vi "iWorx - Spirometer.vi"() -> ()   [LabVIEW 2012]
uses:
  <vilib>/DAQmx/read.llb/DAQmx Read (Analog 1D Wfm NChan 1Samp).vi
  <vilib>/DAQmx/create/channels.llb/DAQmx Create Channel (AI-Voltage-Basic).vi
  <vilib>/DAQmx/configure/timing.llb/DAQmx Timing (Sample Clock).vi
  <vilib>/DAQmx/miscellaneous.llb/DAQmx Fill In Error Info.vi
panel:
  in  "Reset Integral":bool=TRUE
  in  "Set Up":bool
  out "Offset":dbl
  out "Slope":dbl=26.4
  in  "Set SP2":bool
  in  "Set SP1":bool
  in  "Channel":u16(ring) items=["Channel 1", "Channel 2"]
  in  "Calibration Data":T1={"SP1 Voltage"=1.0, "SP2 Voltage"=0.0, "SP1 Pressure"=26.4, "SP2 Pressure"=0.0} {"SP2 Voltage" format="%#_g V"; "SP1 Voltage" format="%#_g V"}
  in  "Pause Button":bool
  in  "Snapshot":bool
  out "Processed Signal":dbl(knob) caption="Pressue (mm H2O)" scale=-200.0..200.0
  in  "stop":bool
  out "Waveform Chart":waveform(dbl)[](graph)
  in  "Clear Chart":bool
  in  "Open Log":bool
  in  "Autoscale Y":bool=TRUE
  out "Raw Signal":dbl(knob) scale=-10.0..10.0
  # "iWorx - Spirometer - Data Logger"
  # "Sensor Input"
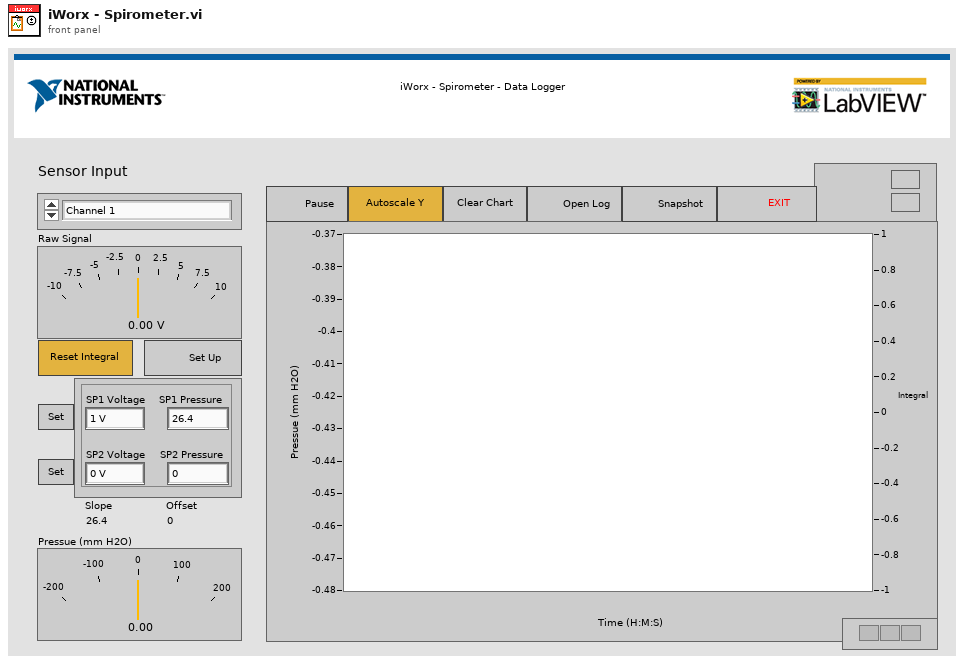
[diagram p1: front panel]
types:
  T1 = cluster{"SP1 Voltage":dbl, "SP2 Voltage":dbl, "SP1 Pressure":dbl, "SP2 Pressure":dbl}
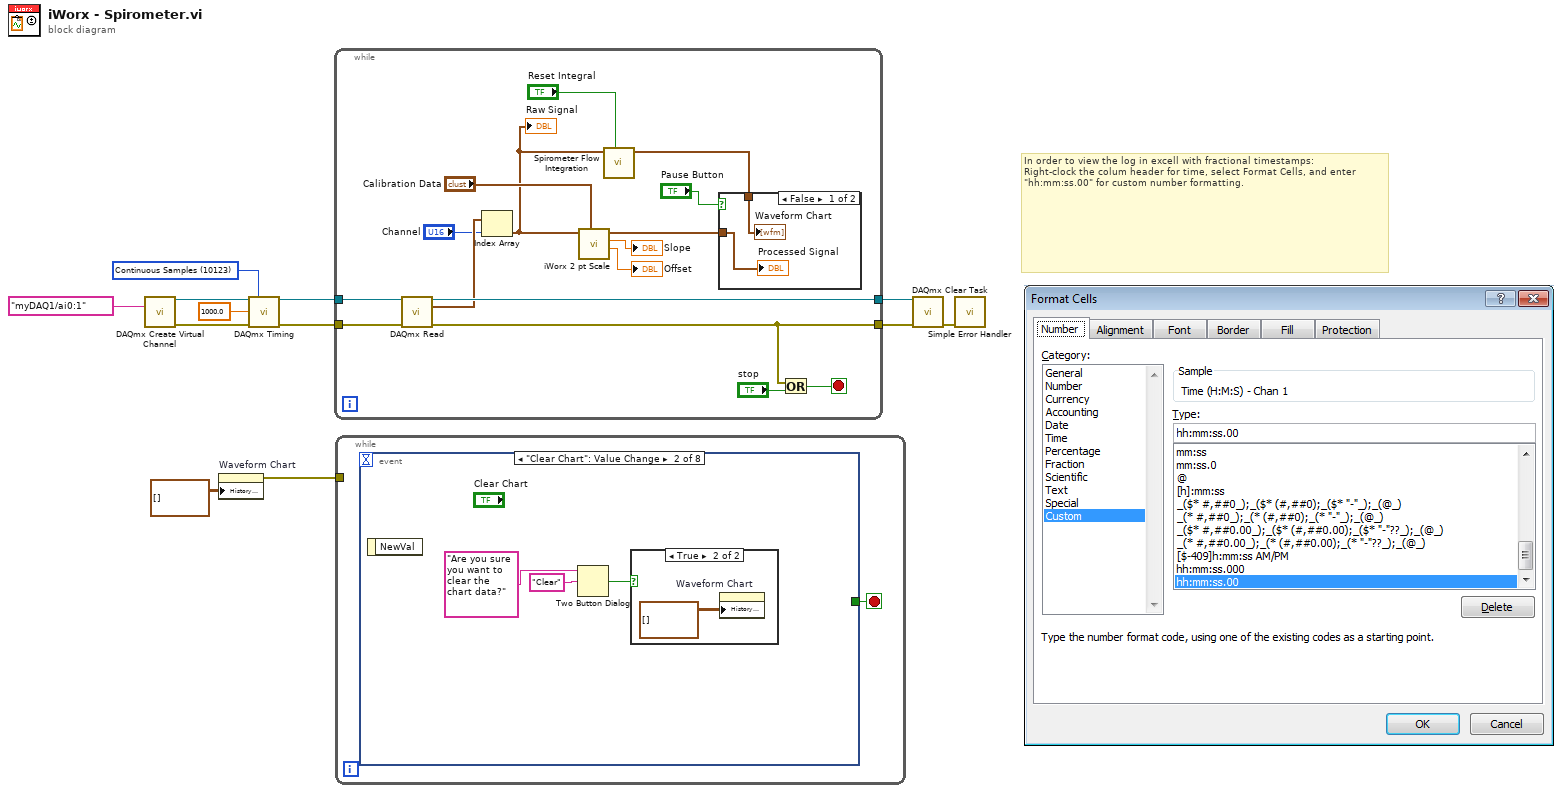
[diagram p0: block diagram]
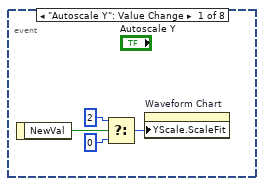
[diagram p2: hidden frame]
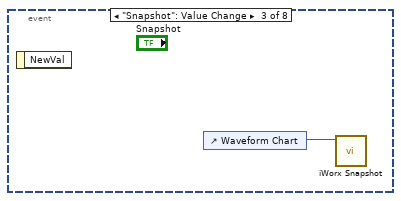
[diagram p4: hidden frame]
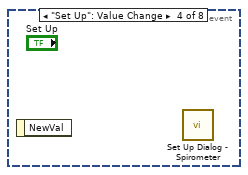
[diagram p5: hidden frame]
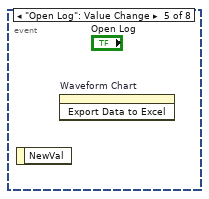
[diagram p6: hidden frame]
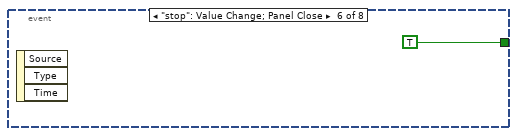
[diagram p7: hidden frame]
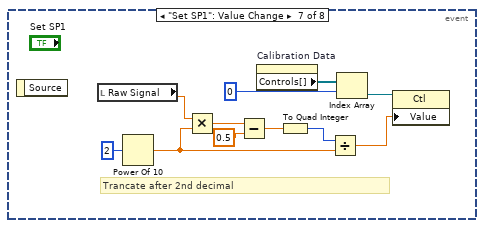
[diagram p8: hidden frame]
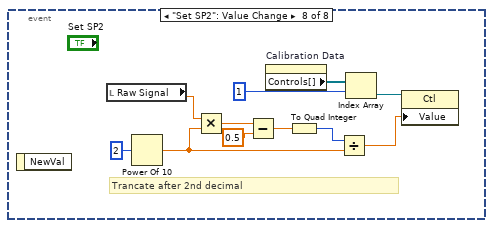
[diagram p9: hidden frame]
diagram:
  w2 = 10123 items=["Finite Samples"=10178, "Continuous Samples"=10123, "Hardware Timed Single Point"=12522] ("sample mode")
  # "In order to view the log in excell with fractional timestamps: \nRight-clock the colum header for time, select Format Cells, and enter \"hh:mm:ss.00\" for custom number formatting."
  n1 = call-poly <vilib>:"DAQmx Create Virtual Channel.vi"("physical channels"=tag "myDAQ1/ai0:1") -> ("task out"=w6:refnum<k21>, "error out"=w5:errorcluster)  [unwired: 13 in]
  n2 = property on="Waveform Chart" class="WFChart (strict)"("History Data"=waveform(dbl)[][] []) -> (error out=w9:errorcluster)  [unwired: 2 in, 1 out]
  n3 = call-poly <vilib>:"DAQmx Timing.vi"("task/channels in"=w6, "sample mode"=w2, "rate"=1000.0, "error in"=w5) -> ("task out"=w4:refnum<k21>, "error out"=w3:errorcluster)  [unwired: 10 in]
  n4 = while {
    tunnel: w4 -> [w27]
    tunnel: [w26] -> w12
    tunnel: w3 -> [w25]
    tunnel: [w23] -> w11
    stop <- w24 stop-if-true
    n5 = call-poly <vilib>:"DAQmx Read.vi"("task/channels in"=w27, "error in"=w25) -> ("task out"=w26:refnum<k21>, "data"=w21:waveform(dbl)[], "error out"=w23:errorcluster)  [unwired: 11 in]
    n6 = Index Array(array=w21, index="Channel") -> (element=w13:waveform(dbl))
    "Raw Signal" <- w13
    n7 = call "iWorx 2 pt Scale.vi"("Set Points"="Calibration Data", "Raw Waveform"=w13) -> ("Offset"=→"Offset":dbl, "Slope"=→"Slope":dbl, "Scaled Value"=w20:waveform(dbl))  [unwired: 7 in]
    n8 = call "Spirometer Flow Integration.vi"("Reset Integral"="Reset Integral", "Waveform in"=w13) -> ("Waveform Array"=w15:waveform(dbl)[])  [unwired: 9 in]
    n9 = case shown="False" "Pause Button" {
      tunnel: w20 -> [w30 _]
      tunnel: w15 -> [w29 _]
      frame False {
        "Waveform Chart" <- w29
        "Processed Signal" <- w30
      }
      frame True {
      }
    }
    n10 = Or(x=w23, y="stop") -> (x .or. y?=w24:bool)
  }
  n11 = while {
    tunnel: w9 -> [_]
    stop <- w31 stop-if-true
    n12 = event shown="[1] \"Clear Chart\": Value Change" {
      selector: _ -> [_ _ _ _ _ _ _ _]
      dyn-events: _ -> [_ _ _ _ _ _ _ _]
      timeout: _ -> [_ _ _ _ _ _ _ _]
      tunnel: [_ _ _ _ _ TRUE _ _] -> w31
      event "Autoscale Y": Value Change {
        n13 = event-data() -> ("NewVal"=w33:bool)  [unwired: 1 in]
        n14 = Select(t=u8 2 ("Y Scale.Scale Fit"), s=w33, f=u8 0 ("Y Scale.Scale Fit")) -> (s? t:f=w32:u8)
        n15 = property on="Waveform Chart" class="WFChart (strict)"("YScale.ScaleFit"=w32) -> ()  [unwired: 2 in, 2 out]
      }
      event "Clear Chart": Value Change {
        n16 = event-data() -> ()  [unwired: 1 in, 1 out]
        n17 = Two Button Dialog(message="Are you sure you want to clear the chart data?", 2:"Clear" ("T button name (\"OK\")")) -> (T button?=w37:bool)  [unwired: 1 in]
        n18 = case shown="True" w37 {
          frame False {
          }
          frame True {
            n19 = property on="Waveform Chart" class="WFChart (strict)"("History Data"=waveform(dbl)[][] []) -> ()  [unwired: 2 in, 2 out]
          }
        }
      }
      event "Snapshot": Value Change {
        n20 = event-data() -> ()  [unwired: 1 in, 1 out]
        n21 = control-ref of="Waveform Chart"() -> (w40:refnum<vi>)
        n22 = call "iWorx Snapshot.vi"("WaveformChart in"=w40) -> ()  [unwired: 10 in, 1 out]
      }
      event "Set Up": Value Change {
        n23 = event-data() -> ()  [unwired: 1 in, 1 out]
        n24 = call "Set Up Dialog - Spirometer.vi"() -> ()  [unwired: 12 in]
      }
      event "Open Log": Value Change {
        n25 = event-data() -> ()  [unwired: 1 in, 1 out]
        n26 = invoke on="Waveform Chart" class="WFChart (strict)" method="Export Data to Excel"() -> ()  [unwired: 3 in, 3 out]
      }
      event "stop": Value Change; Panel Close {
        n27 = event-data() -> ()  [unwired: 1 in, 3 out]
      }
      event "Set SP1": Value Change {
        # "Trancate after 2nd decimal"
        n28 = event-data() -> ()  [unwired: 1 in, 1 out]
        n29 = local read "Raw Signal"() -> (w42:dbl)
        n30 = Power Of 10(x=2) -> (10^x=w49:dbl)
        n31 = Multiply(x=w42, y=w49) -> (x*y=w47:dbl)
        n32 = Subtract(x=w47, y=0.5) -> (x-y=w46:dbl)
        n33 = property on="Calibration Data" class="Clust (strict)"() -> ("Controls[]"=w52:refnum<vi>[])  [unwired: 2 in, 2 out]
        n34 = To Quad Integer(1:w46) -> (0:w48:i64)
        n35 = Divide(x=w48, y=w49) -> (x/y=w44:dbl)
        n36 = Index Array(array=w52, index=0) -> (element=w51:refnum<vi>)
        n37 = property class="Ctl"(reference=w51, "Value"=w44) -> ()  [unwired: 1 in, 2 out]
      }
      event "Set SP2": Value Change {
        # "Trancate after 2nd decimal"
        n38 = event-data() -> ()  [unwired: 1 in, 1 out]
        n39 = local read "Raw Signal"() -> (w53:dbl)
        n40 = Power Of 10(x=2) -> (10^x=w60:dbl)
        n41 = Multiply(x=w53, y=w60) -> (x*y=w58:dbl)
        n42 = Subtract(x=w58, y=0.5) -> (x-y=w57:dbl)
        n43 = property on="Calibration Data" class="Clust (strict)"() -> ("Controls[]"=w63:refnum<vi>[])  [unwired: 2 in, 2 out]
        n44 = To Quad Integer(1:w57) -> (0:w59:i64)
        n45 = Divide(x=w59, y=w60) -> (x/y=w55:dbl)
        n46 = Index Array(array=w63, index=1) -> (element=w62:refnum<vi>)
        n47 = property class="Ctl"(reference=w62, "Value"=w55) -> ()  [unwired: 1 in, 2 out]
      }
    }
  }
  n48 = call <vilib>:"DAQmx Clear Task.vi"("task in"=w12, "error in"=w11) -> ("error out"=w8:errorcluster)  [unwired: 13 in]
  n49 = call <vilib>:"Simple Error Handler.vi"("error in (no error)"=w8) -> ()  [unwired: 4 in, 5 out]
